vi "Create.vi"(7 "Size":i32, 8 "error in (no error)":errorcluster, 10 "Channel Info":T1) -> (0 "error out":errorcluster, 3 "Channel Buffer DBL out":refnum<class "Channel Buffer DBL.lvclass">)   [LabVIEW 2020, in "VolatusHistorian.lvlib" / "Channel Buffer DBL.lvclass"]
uses:
  Channel Buffer DBL.lvclass
  Channel Buffer DBL.lvclass/Channel Buffer DBL.ctl
  lv-vecto/Vecto/Channel Info.ctl
  lv-vecto/VectoConfig/VectoConfig.lvlib
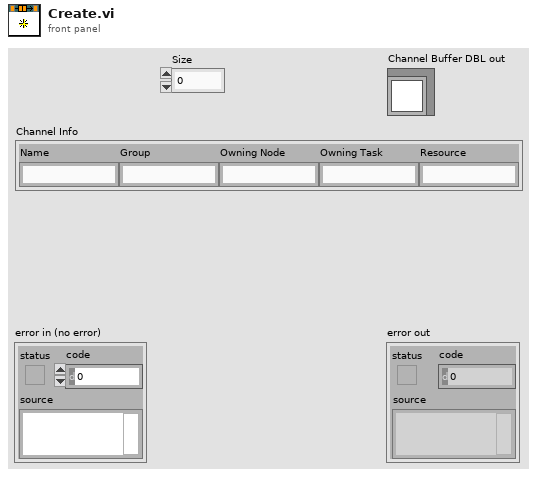
[diagram p1: front panel]
types:
  T1 = typedef "VectoConfig.lvlib/Channel Info.ctl" = cluster{"Name":string, "Group":string, "Owning Node":string, "Owning Task":string, "Resource":string}
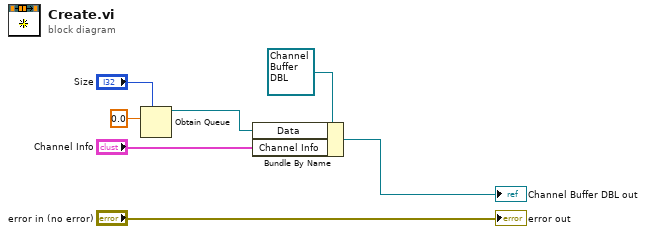
[diagram p0: block diagram]
diagram:
  n1 = Obtain Queue(max queue size (-1, unlimited)="Size", element data type=0.0) -> (queue out=w2:refnum<queue>)  [unwired: 3 in, 2 out]
  n2 = Bundle By Name(cluster=refnum<class "Channel Buffer DBL.lvclass"> refnum ("Channel Buffer DBL in"), "Data"=w2, "Channel Info"="Channel Info") -> (→"Channel Buffer DBL out":refnum<class "Channel Buffer DBL.lvclass">)
  "error out" <- "error in (no error)"
